vi "MAV_CMD_DO_CHANGE_SPEED.vi"(9 "Throttle(%)":sgl=-1.0, 10 "Speed(m/s)":sgl=-1.0, 11 "Ground Speed(T)/Airspeed(F)":bool) -> (3 "MAVLink Message":u8[](array[numeric]))   [LabVIEW 2014]
panel:
  out "Payload Size":i32
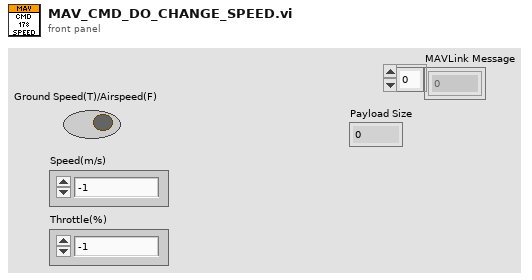
[diagram p1: front panel]
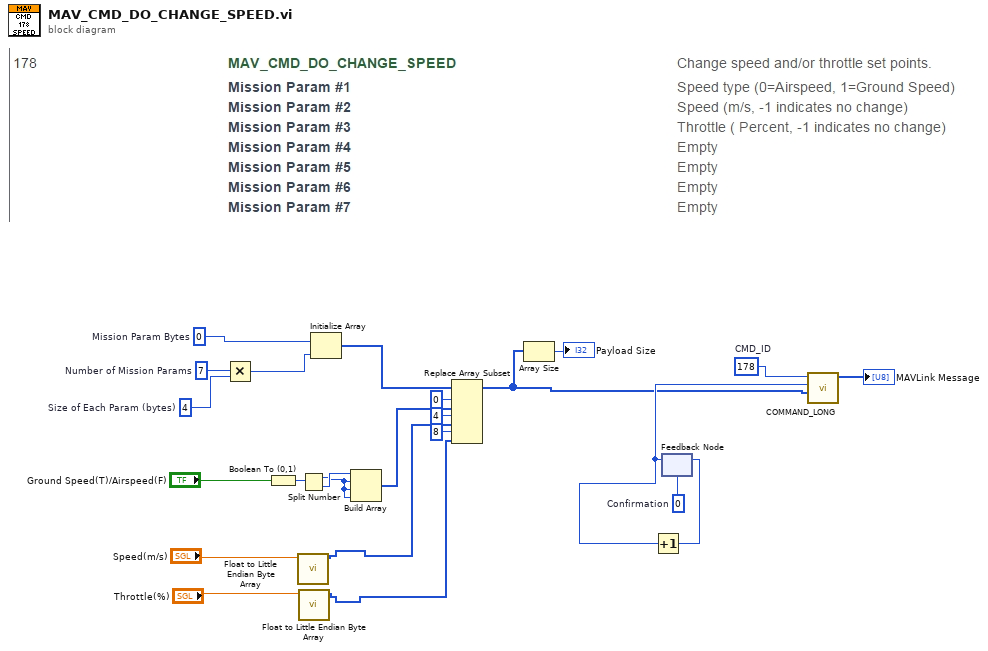
[diagram p0: block diagram]
diagram:
  w10 = u8 0  # Confirmation
  w21 = 4  # Size of Each Param (bytes)
  w22 = 7  # Number of Mission Params
  w23 = u8 0  # Mission Param Bytes
  w8 = u16 178  # CMD_ID
  n1 = Multiply(x=w22, y=w21) -> (x*y=w20:i32)
  n2 = Boolean To (0,1)(Boolean="Ground Speed(T)/Airspeed(F)") -> (0, 1=w19:i16)
  n3 = call "Float to Little Endian Byte Array.vi"("Float In"="Speed(m/s)") -> ("LE Byte Array"=w5:u8[])  [unwired: 10 in]
  n4 = Split Number(x=w19) -> (hi(x)=w17:u8, lo(x)=w18:u8)
  n5 = call "Float to Little Endian Byte Array.vi"("Float In"="Throttle(%)") -> ("LE Byte Array"=w4:u8[])  [unwired: 10 in]
  n6 = Initialize Array(w23, w20) -> (w16:u8[])
  n7 = Build Array(w18, w17, w17, w17) -> (w12:u8[])
  n8 = Replace Array Subset(array=w16, new element #1=w12, index #1=0 ("index"), new element #2=w5, index #2=4 ("index"), new element #3=w4, index #3=8 ("index")) -> (w6:u8[])
  n9 = Array Size(array=w6) -> (size(s)=→"Payload Size":i32)
  n10 = feedback #1(w10) -> (w7:u8)
  n11 = Increment(x=w7) -> (x+1=w9:u8)
  n12 = feedback-in #1(w9) -> ()
  n13 = call "COMMAND_LONG.vi"("Mission Params"=w6, "Confirmation"=w7, "Command ID"=w8) -> ("MAVLink Message"=→"MAVLink Message":u8[])  [unwired: 8 in]
